vi "1B_HiStim_BuildTriggerArray.vi"(0 "CBC Trigger Level":dbl, 1 "Load Resistance (Ohms)":dbl, 2 "Target Stim Current (Amps)":dbl, 3 "Krec Value":i32, 4 "Recovery Mode (T=Active)":bool) -> (5 "Pulse Triggers":T1(array[cluster]))   [LabVIEW 2010]
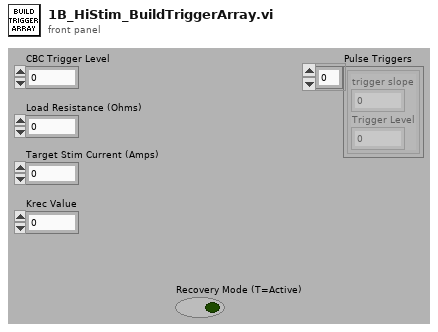
[diagram p1: front panel]
types:
  T1 = cluster{"trigger slope":u16, "Trigger Level":dbl}[]
  T2 = cluster{"trigger slope":u16, "Trigger Level":dbl}
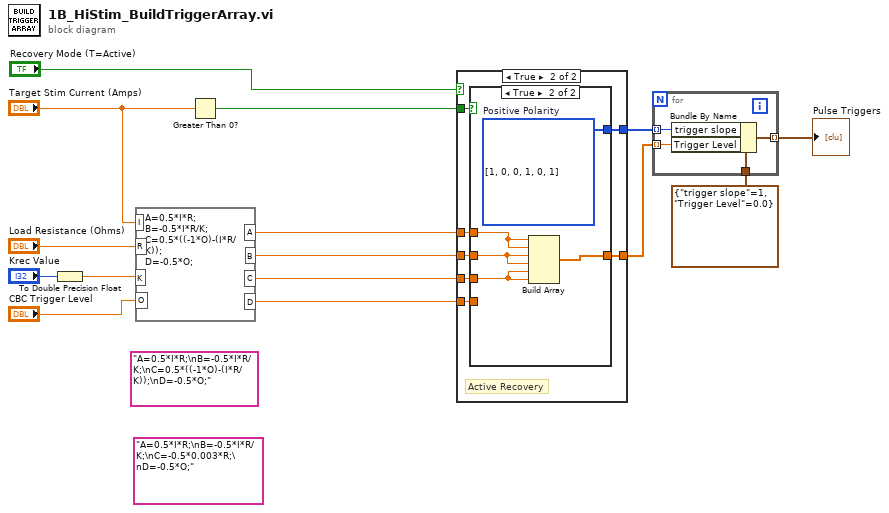
[diagram p0: block diagram]
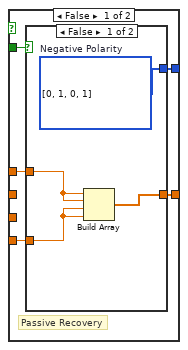
[diagram p2: hidden frame]
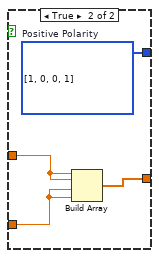
[diagram p3: hidden frame]
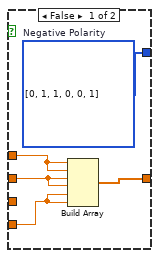
[diagram p4: hidden frame]
diagram:
  (unwired) "A=0.5*I*R;\nB=-0.5*I*R/K;\nC=-0.5*0.003*R;\nD=-0.5*O;"
  (unwired) "A=0.5*I*R;\nB=-0.5*I*R/K;\nC=0.5*((-1*O)-(I*R/K));\nD=-0.5*O;"
  n1 = To Double Precision Float(number="Krec Value") -> (double precision float=w8:dbl)
  n2 = formula code="A=0.5*I*R;\nB=-0.5*I*R/K;\nC=0.5*((-1*O)-(I*R/K));\nD=-0.5*O;"("R"="Load Resistance (Ohms)", "I"="Target Stim Current (Amps)", "K"=w8, "O"="CBC Trigger Level") -> ("A"=w5:dbl, "B"=w4:dbl, "C"=w3:dbl, "D"=w2:dbl)
  n3 = Greater Than 0?(x="Target Stim Current (Amps)") -> (x > 0?=w14:bool)
  n4 = case shown="True" "Recovery Mode (T=Active)" {
    tunnel: [w19 w35] -> w11
    tunnel: w14 -> [w20 w34]
    tunnel: w5 -> [w18 w33]
    tunnel: w4 -> [_ w32]
    tunnel: w3 -> [_ w31]
    tunnel: w2 -> [w17 w30]
    tunnel: [w16 w29] -> w1
    frame False {
      # "Passive Recovery"
      n5 = case shown="False" w20 {
        tunnel: [w24 w28] -> w19
        tunnel: w18 -> [w23 w27]
        tunnel: w17 -> [w22 w26]
        tunnel: [w21 w25] -> w16
        frame False {
          w24 = u16[] [0, 1, 0, 1] items=["Falling Edge", "Rising Edge"]  # Negative Polarity
          n6 = Build Array(w23, w23, w22, w22) -> (w21:dbl[])
        }
        frame True {
          w28 = u16[] [1, 0, 0, 1] items=["Falling Edge", "Rising Edge"]  # Positive Polarity
          n7 = Build Array(w27, w27, w26, w26) -> (w25:dbl[])
        }
      }
    }
    frame True {
      # "Active Recovery"
      n8 = case shown="True" w34 {
        tunnel: [w40 w45] -> w35
        tunnel: w33 -> [w39 w44]
        tunnel: w32 -> [w37 w41]
        tunnel: w31 -> [_ w42]
        tunnel: w30 -> [w36 _]
        tunnel: [w38 w43] -> w29
        frame False {
          w40 = u16[] [0, 1, 1, 0, 0, 1] items=["Falling Edge", "Rising Edge"]  # Negative Polarity
          n9 = Build Array(w39, w39, w37, w37, w36, w36) -> (w38:dbl[])
        }
        frame True {
          w45 = u16[] [1, 0, 0, 1, 0, 1] items=["Falling Edge", "Rising Edge"]  # Positive Polarity
          n10 = Build Array(w44, w44, w41, w41, w42, w42) -> (w43:dbl[])
        }
      }
    }
  }
  n11 = for {
    tunnel: T2 {"trigger slope"=1, "Trigger Level"=0.0} -> [w49]
    tunnel: w11 -> [w48] mode=indexing
    tunnel: w1 -> [w47] mode=indexing
    tunnel: [w46] -> w13 mode=indexing
    n12 = Bundle By Name(cluster=w49, "trigger slope"=w48, "Trigger Level"=w47) -> (w46:T2)
  }
  "Pulse Triggers" <- w13
